vi "4_1.vi"() -> ()   [LabVIEW 2023]
panel:
  in  "stop":bool
  out "Numeric":dbl
  out "Meter":dbl(knob) scale=0.0..10000.0
  out "Waveform Graph":dynamicdata(graph)
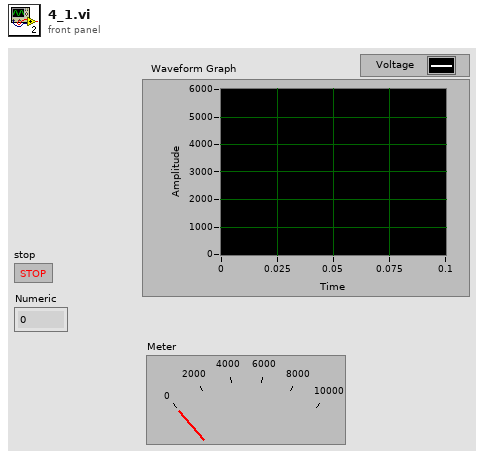
[diagram p1: front panel]
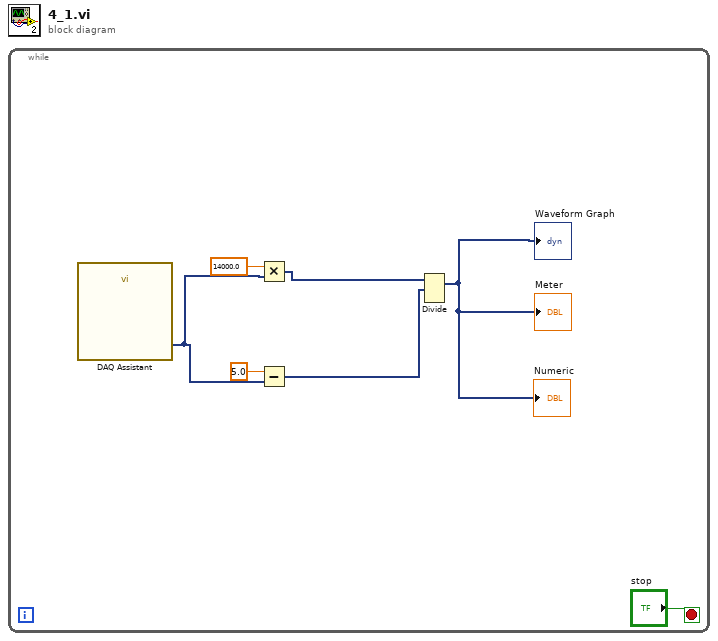
[diagram p0: block diagram]
diagram:
  n1 = while {
    stop <- "stop" stop-if-true
    n2 = call "DAQ Assistant"() -> ("data"=w7:dynamicdata)  [unwired: 17 in, 2 out]
    n3 = Multiply(x=14000.0, y=w7) -> (x*y=w4:dynamicdata)
    n4 = Subtract(x=5.0, y=w7) -> (x-y=w3:dynamicdata)
    n5 = Divide(1:w3, 2:w4) -> (0:→"Waveform Graph" →"Meter" →"Numeric":dynamicdata)  [unwired: 1 in, 1 out]
  }
